vi "Zero Force Test.vi"(8 "error in (no error)":errorcluster, 10 "Model in":refnum<class "Model.lvclass">, 11 "Test Actuator State in":refnum<class "Test Actuator State.lvclass">) -> (0 "error out":errorcluster, 2 "Model out":refnum<class "Model.lvclass">, 3 "Test Actuator State out":refnum<class "Test Actuator State.lvclass">)   [LabVIEW 2016]
uses:
  Model/Model/Model.lvclass
  Typedefs/ActuatorSetPoints.ctl
  <vilib>/platform/TimedLoop/XDataNode/XDataNode.xnode
  <vilib>/Platform/TimedLoop/XDataNode/nitl_modes.ctl
  <vilib>/Platform/TimedLoop/XDataNode/XDNodeRunTimeDep.lvlib
  <vilib>/Platform/TimedLoop/XDataNode/wakeup.ctl
  <vilib>/Platform/TimedLoop/XDataNode/timing_clust.ctl
  Typedefs/TestStatus.ctl
  Typedefs/HPMT_Typedefs.lvlib
  Test Actuator State.lvclass
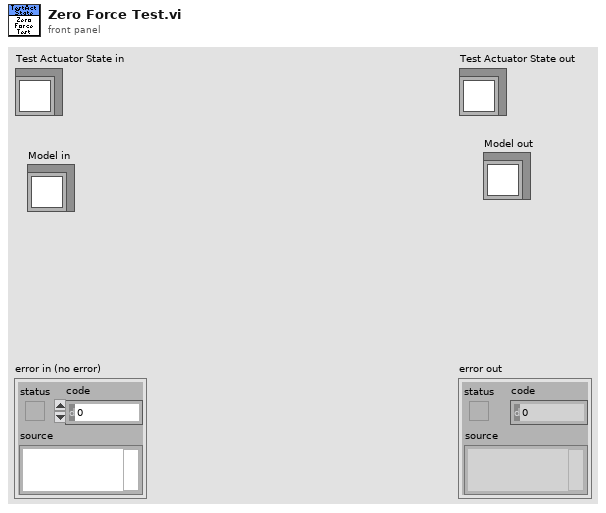
[diagram p1: front panel]
types:
  T1 = typedef "HPMT_Typedefs.lvlib/TestStatus.ctl" = enum16{"Not Run", "Running", "Passed", "Failed"}
  T2 = typedef "ActuatorSetPoints.ctl" = cluster{"Axial Force":dbl, "Lateral Force":dbl, "FC1 Force":dbl, "FC2 Force":dbl}
  T3 = typedef "HPMT_Typedefs.lvlib/AllTestStatus.ctl" = cluster{"Test One":T1}
  T4 = typedef "XDNodeRunTimeDep.lvlib/timing_clust.ctl" = cluster{"Expected End [f-1]":u64, "Actual End [f-1]":u64, "Finished Late? [f-1]":bool, "Expected End [i-1]":u64, "Actual End [i-1]":u64, "Finished Late? [i-1]":bool, "Expected Start [i]":u64, "Actual Start [i]":u64, "Expected Start [f]":u64, "Actual Start [f]":u64, "Source Name":string, "Structure Name":string, "Period":i64, "Deadline":i64, "Offset":i64, "Start":i64, "Priority":i32, "Timeout":i32, "Mode":T5, "Wakeup Reason":T6, "Error":errorcluster, "Source Type":string, "Secondary Source Type":string, "Global End Time":u64, "Global Start Time":u64, "Frame Duration":u64, "Iteration Duration":u64, "Assigned CPU":i32, "I/O Scan Engine Mode":u32}
  T5 = typedef "XDNodeRunTimeDep.lvlib/nitl_modes.ctl" = enum32{"No Change", "Process missed periods, maintain original phase", "Discard missed periods, maintain original phase", "Process missed periods, ignore original phase", "Discard missed periods, ignore original phase"}
  T6 = typedef "XDNodeRunTimeDep.lvlib/wakeup.ctl" = enum32{"Normal", "Aborted", "Asynchronous wakeup", "Timing source error", "Timed loop error", "Timeout"}
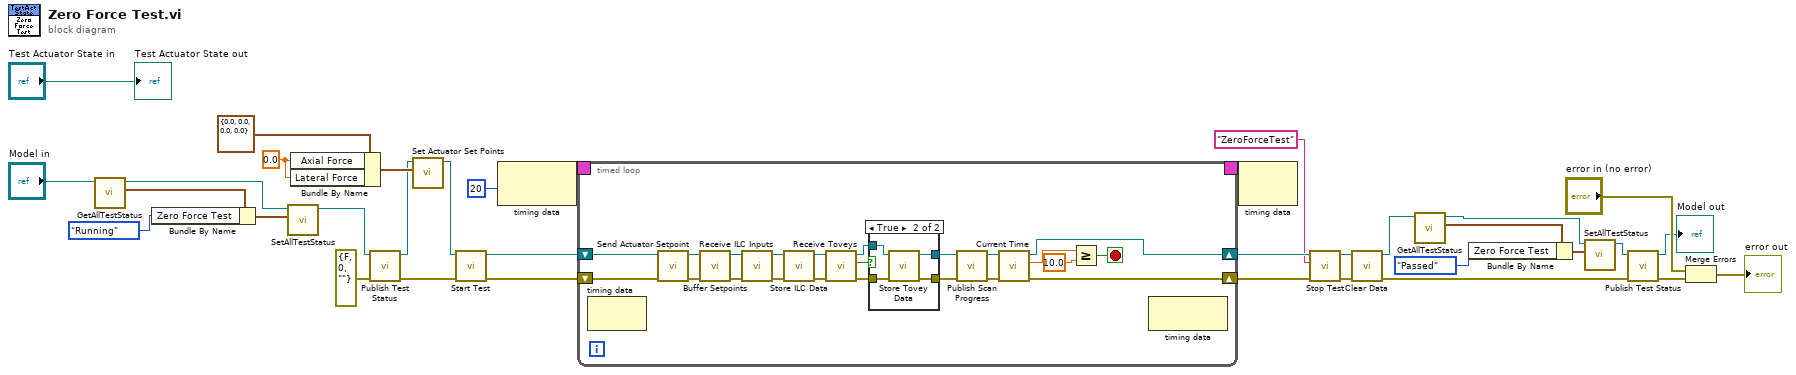
[diagram p0: block diagram]
diagram:
  w21 = 0.0 ("Axial Force")
  n1 = call "GetAllTestStatus.vi"("Model in"="Model in") -> ("AllTestStatus"=w15:T3, "Model out"=w18:refnum<class "Model.lvclass">)  [unwired: 9 in]
  n2 = Bundle By Name(cluster=w15, "Zero Force Test"=TestStatus."Running" ("Full Force Test")) -> (w16:T3)
  n3 = call "SetAllTestStatus.vi"("AllTestStatus"=w16, "Model in"=w18) -> ("Model out"=w13:refnum<class "Model.lvclass">)  [unwired: 9 in]
  n4 = Bundle By Name(cluster=T2 {"Axial Force"=0.0, "Lateral Force"=0.0, "FC1 Force"=0.0, "FC2 Force"=0.0} ("Actuator Set Points"), "Axial Force"=w21, "Lateral Force"=w21) -> (w29:T2)
  n5 = call "Publish Test Status.vi"("error in (no error)"=errorcluster {"status"=FALSE, "code"=0, "source"=""} ("error out"), "Model in"=w13) -> ("error out"=w10:errorcluster, "Model out"=w12:refnum<class "Model.lvclass">)  [unwired: 8 in]
  n6 = call "Set Actuator Set Points.vi"("Actuator Set Points"=w29, "Model in"=w12) -> ("Model out"=w26:refnum<class "Model.lvclass">)  [unwired: 9 in]
  n7 = call "Start Test.vi"("error in (no error)"=w10, "Model in"=w26) -> ("error out"=w27:errorcluster, "Model out"=w25:refnum<class "Model.lvclass">)  [unwired: 8 in]
  n8 = node-c288(i64 20 ("Period")) -> (w32:T4)
  n9 = timed-loop {
    shift-right: [w53] -> w24
    shift-left: w25 -> [w57]
    shift-right: [w52] -> w23
    shift-left: w27 -> [w55]
    timing: w32 -> [_]
    timing-out: [_] -> w31
    stop <- w50 stop-if-true
    n10 = node-c288() -> ()  [unwired: 1 in, 1 out]
    n11 = call "Send Actuator Setpoint.vi"("error in (no error)"=w55, "Model in"=w57) -> ("error out"=w38:errorcluster, "Model out"=w40:refnum<class "Model.lvclass">)  [unwired: 8 in]
    n12 = call "Buffer Setpoints.vi"("error in (no error)"=w38, "Model in"=w40) -> ("error out"=w37:errorcluster, "Model out"=w39:refnum<class "Model.lvclass">)  [unwired: 8 in]
    n13 = call "Receive ILC Inputs.vi"("error in (no error)"=w37, "Model in"=w39) -> ("error out"=w54:errorcluster, "Model out"=w56:refnum<class "Model.lvclass">)  [unwired: 8 in]
    n14 = call "Store ILC Data.vi"("error in (no error)"=w54, "Model in"=w56) -> ("error out"=w48:errorcluster, "Model out"=w49:refnum<class "Model.lvclass">)  [unwired: 8 in]
    n15 = call "Receive Toveys.vi"("error in (no error)"=w48, "Model in"=w49) -> ("error out"=w46:errorcluster, "Data Received"=w45:bool, "Model out"=w47:refnum<class "Model.lvclass">)  [unwired: 7 in]
    n16 = case shown="True" w45 {
      tunnel: w47 -> [w61 w65]
      tunnel: w46 -> [w60 w64]
      tunnel: [w60 w63] -> w41
      tunnel: [w61 w62] -> w44
      frame False {
      }
      frame True {
        n17 = call "Store Tovey Data.vi"("error in (no error)"=w64, "Model in"=w65) -> ("error out"=w63:errorcluster, "Model out"=w62:refnum<class "Model.lvclass">)  [unwired: 8 in]
      }
    }
    n18 = call "Publish Scan Progress.vi"("error in (no error)"=w41, "Model in"=w44) -> ("error out"=w42:errorcluster, "Model out"=w43:refnum<class "Model.lvclass">)  [unwired: 8 in]
    n19 = call "Current Time.vi"("error in (no error)"=w42, "Model in"=w43) -> ("error out"=w52:errorcluster, "Time"=w51:dbl, "Model out"=w53:refnum<class "Model.lvclass">)  [unwired: 7 in]
    n20 = Greater Or Equal?(x=w51, y=10.0) -> (x >= y?=w50:bool)
    n21 = node-c288() -> ()  [unwired: 1 in, 1 out]
  }
  n22 = node-c288(w31) -> ()  [unwired: 1 out]
  n23 = call "Stop Test.vi"("error in (no error)"=w23, "Test"="ZeroForceTest", "Model in"=w24) -> ("error out"=w19:errorcluster, "Model out"=w20:refnum<class "Model.lvclass">)  [unwired: 7 in]
  n24 = call "Clear Data.vi"("error in (no error)"=w19, "Model in"=w20) -> ("error out"=w3:errorcluster, "Model out"=w5:refnum<class "Model.lvclass">)  [unwired: 8 in]
  n25 = call "GetAllTestStatus.vi"("Model in"=w5) -> ("AllTestStatus"=w6:T3, "Model out"=w8:refnum<class "Model.lvclass">)  [unwired: 9 in]
  n26 = Bundle By Name(cluster=w6, "Zero Force Test"=TestStatus."Passed") -> (w7:T3)
  n27 = call "SetAllTestStatus.vi"("AllTestStatus"=w7, "Model in"=w8) -> ("Model out"=w9:refnum<class "Model.lvclass">)  [unwired: 9 in]
  n28 = call "Publish Test Status.vi"("error in (no error)"=w3, "Model in"=w9) -> ("error out"=w2:errorcluster, "Model out"=→"Model out":refnum<class "Model.lvclass">)  [unwired: 8 in]
  n29 = Merge Errors("error in (no error)", w2) -> (→"error out":errorcluster)
  "Test Actuator State out" <- "Test Actuator State in"
